vi "Parse Gold Board File.vi"(8 "error in (no error)":errorcluster, 11 "Golden Board in":refnum<class "Golden Board.lvclass">) -> (0 "error out":errorcluster, 3 "Golden Board out":refnum<class "Golden Board.lvclass">)   [LabVIEW 2017, in "Golden Board.lvlib" / "Golden Board.lvclass"]
doc: "Loads a gold board file at \"Gold Board File Path\". This method only works for gold boards files used up until TBD. Files created after this date should use the newer method."
uses:
  Golden Board.lvclass
  <vilib>/regexp/Match Regular Expression.xnode
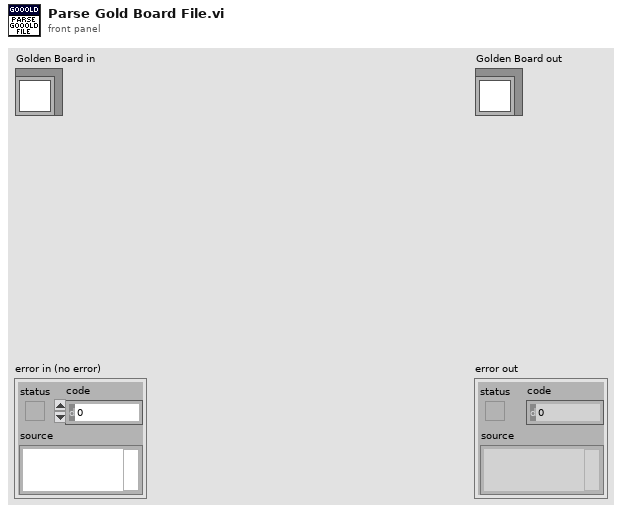
[diagram p1: front panel]
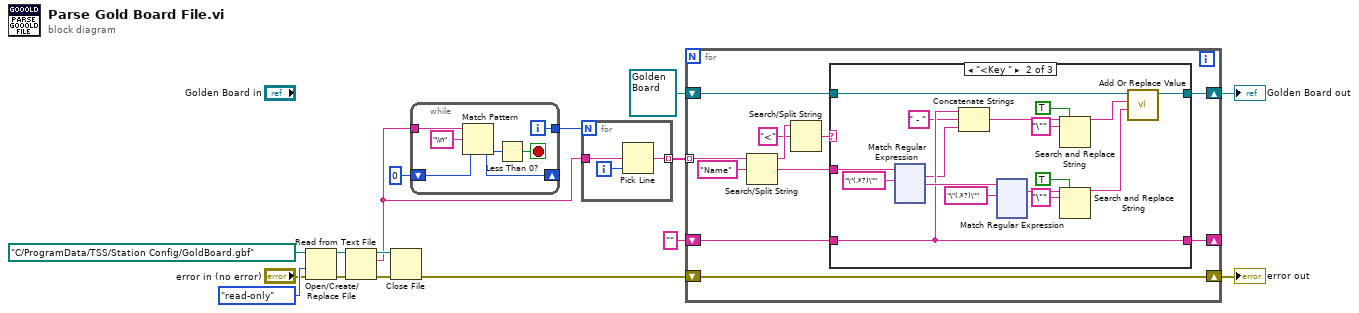
[diagram p0: block diagram]
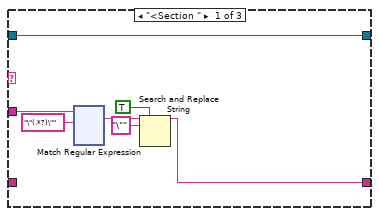
[diagram p2: hidden frame]
diagram:
  n1 = Open/Create/Replace File(file path (use dialog)=path "C:/ProgramData/TSS/Station Config/GoldBoard.gbf", error in="error in (no error)", access (0:read/write)=enum16{"read/write", "read-only", "write-only"}."read-only") -> (refnum out=w14:refnum<file>, error out=w11:errorcluster)  [unwired: 3 in, 1 out]
  n2 = Read from Text File(file (use dialog)=w14, error in=w11) -> (refnum out=w13:refnum<file>, text=w7:string, error out=w12:errorcluster)  [unwired: 2 in, 1 out]
  n3 = Close File(refnum=w13, error in=w12) -> (error out=w3:errorcluster)  [unwired: 1 out]
  n4 = while {
    tunnel: [w21] -> w8
    shift-right: [w19] -> _
    shift-left: 0 ("offset past match") -> [w18]
    tunnel: w7 -> [w17]
    i -> [w21]
    stop <- w20 stop-if-true
    n5 = Match Pattern(string=w17, regular expression="\\n", offset (0)=w18) -> (offset past match=w19:i32)  [unwired: 3 out]
    n6 = Less Than 0?(x=w19) -> (x < 0?=w20:bool)
  }
  n7 = for {
    N: w8 -> [_]
    tunnel: w7 -> [w24]
    tunnel: [w23] -> w6 mode=indexing
    i -> [w25]
    n8 = Pick Line(multi-line string=w24, line index=w25) -> (output string=w23:string)  [unwired: 1 in]
  }
  n9 = for {
    shift-right: [w31] -> _
    shift-left: "" -> [w32]
    shift-right: [w35] -> w10
    shift-left: refnum<class "Golden Board.lvclass"> refnum ("Registry out") -> [w36]
    tunnel: w6 -> [w34] mode=indexing
    shift-right: [w26] -> w4
    shift-left: w3 -> [w26]
    n10 = Search/Split String(string=w34, search string/char (-)="Name") -> (substring before match=w29:string, match + rest of string=w30:string)  [unwired: 1 in, 1 out]
    n11 = Search/Split String(string=w29, search string/char (-)="<") -> (match + rest of string=w28:string)  [unwired: 1 in, 2 out]
    n12 = case shown="\"<Key \"" w28 {
      tunnel: w36 -> [w43 w174 w404]
      tunnel: [w43 w173 w404] -> w35
      tunnel: w32 -> [_ w168 w403]
      tunnel: [w37 w168 w403] -> w31
      tunnel: w30 -> [w42 w171 _]
      frame "<Section " {
        n13 = xnode "Match Regular Expression"("input string"=w42, "regular expression"="\"(.*?)\"") -> ("whole match"=w40:string)  [unwired: 4 in, 4 out]
        n14 = Search and Replace String(replace all?=TRUE ("replace all? (F)"), input string=w40, search string="\"") -> (result string=w37:string)  [unwired: 5 in, 3 out]
      }
      frame "<Key " {
        n15 = xnode "Match Regular Expression"("input string"=w171, "regular expression"="\"(.*?)\"") -> ("whole match"=w167:string, "after match"=w169:string)  [unwired: 4 in, 3 out]
        n16 = Concatenate Strings(w168, " - ", w167) -> (w163:string)
        n17 = xnode "Match Regular Expression"("input string"=w169, "regular expression"="\"(.*?)\"") -> ("whole match"=w159:string)  [unwired: 4 in, 4 out]
        n18 = Search and Replace String(replace all?=TRUE ("replace all? (F)"), input string=w163, search string="\"") -> (result string=w162:string)  [unwired: 5 in, 3 out]
        n19 = Search and Replace String(replace all?=TRUE ("replace all? (F)"), input string=w159, search string="\"") -> (result string=w158:string)  [unwired: 5 in, 3 out]
        n20 = call-dynamic "Add Or Replace Value.vi"("Value"=w158, "Key"=w162, "Registry in"=w174) -> ("Registry out"=w173:refnum<class "Golden Board.lvclass">)  [unwired: 6 in, 2 out]
      }
      frame Default {
      }
    }
  }
  "error out" <- w4
  "Golden Board out" <- w10
